vi "Eliminated.vi"(6 "Column":i32, 8 "Row":i32, 9 "Killer":i32, 10 "Team":i32, 11 "Assassin in":refnum<class "Assassin.lvclass">) -> (3 "Assassin out":refnum<class "Assassin.lvclass">)   [LabVIEW 2015, in "Assassin.lvclass"]
uses:
  Assassin.lvclass
  Square/Square.lvclass
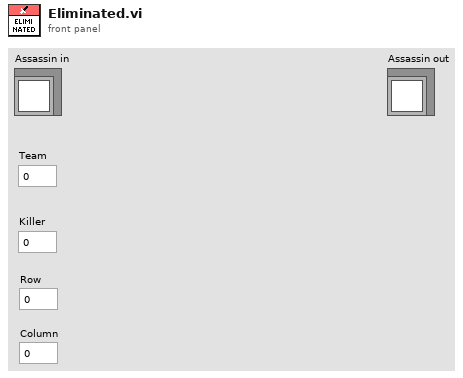
[diagram p1: front panel]
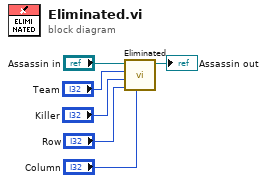
[diagram p0: block diagram]
diagram:
  n1 = call-parent "Eliminated.vi"("Column"="Column", "Row"="Row", "Killer"="Killer", "Team"="Team", "Square in"="Assassin in") -> ("Square out"=→"Assassin out":refnum<class "Assassin.lvclass">)  [unwired: 6 in]
